vi "Setup Connection.vi"(0 "WAMP Client in":refnum<class "WAMP Client.lvclass">, 1 "ICommHandler.lvclass":refnum<class "ICommHandler.lvclass">, 7 "Realm":string, 9 "Address":string, 11 "error in (no error)":errorcluster) -> (4 "WAMP Client out":refnum<class "WAMP Client.lvclass">, 15 "error out":errorcluster)   [LabVIEW 2020, in "wamplv.lvlib" / "WAMP Client.lvclass"]
uses:
  WAMP Client.lvclass
  Private/Comm Handlers/ICommHandler/ICommHandler.lvclass
  WAMP Client.lvclass/WAMP Client.ctl
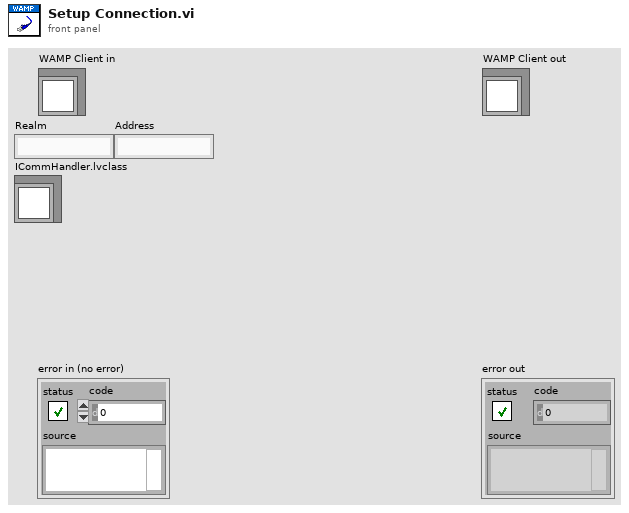
[diagram p1: front panel]
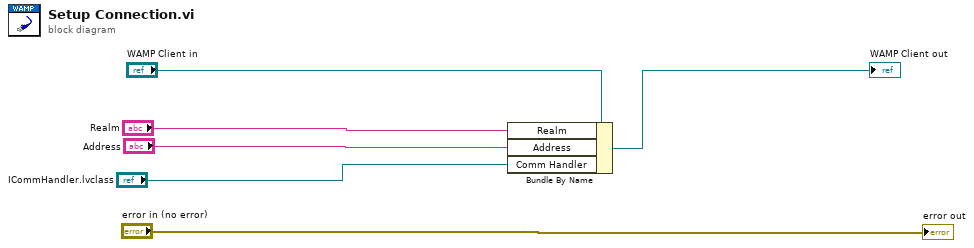
[diagram p0: block diagram]
diagram:
  n1 = Bundle By Name(cluster="WAMP Client in", "Realm"="Realm", "Address"="Address", "Comm Handler"="ICommHandler.lvclass") -> (→"WAMP Client out":refnum<class "WAMP Client.lvclass">)
  "error out" <- "error in (no error)"
